vi "Pauli-Z.vi"   [LabVIEW 2020]
doc: "Pauli-Z Gate\n\nApplies the Phase Flip. \nLeaves |0> unchanged and maps |1> to -|1>. \nRotates by pi radians around the Z-axis. \n\nMatrix: [[ 1, 0], [ 0, -1]]"
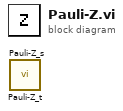
[diagram p0: block diagram]
diagram:
  n1 = call "Pauli-Z_t.vi"() -> ()  [unwired: 15 in, 1 out]
  n2 = call "Pauli-Z_s.vi"() -> ()  [unwired: 15 in, 1 out]
